vi "grabber fpga details panel.vi"() -> ()   [LabVIEW 2010]
uses:
  scan_specification_tagResonant.ctl
  common_typedefs/DAC_voltage_tagResonantr.ctl
  counter_cluster_tagResonant.ctl
  FPGA_ref.ctl
  <vilib>/Platform/TimedLoop/XDataNode/XDataNode.xnode
  <vilib>/Platform/TimedLoop/XDataNode/timing_clust.ctl
  <vilib>/Platform/TimedLoop/XDataNode/nitl_modes.ctl
  <vilib>/Platform/TimedLoop/XDataNode/wakeup.ctl
  <vilib>/rvi/interface/nirviReadWriteControl/nirviReadWriteControl.xnode
  <vilib>/rvi/interface/common/niFpgaNodeNameForErrorReporting.ctl
  <vilib>/rvi/errors/niLvFpgaWhatHappensToTopLevelVI.ctl
  <vilib>/Utility/error.llb/Error Cluster From Error Code.vi
  <vilib>/rvi/errors/niLvFpgaAdjustHostInterfaceError.vi
  <vilib>/Platform/TimedLoop/XDataNode/XDNodeRunTimeDep.lvlib
  NiFpgaLv.dll
panel:
  out "z-location":i16
  out "z state.pos estimate":fxp<+/-,32,16> format="%.21g"
  out "piezo z-offset":i16
  out "piezo out":i16
  in  "FPGARef":T1
  out "counter cluster out":T2
  out "scanning? FPGA":bool
  out "scan":bool
  out "FIFO overflow":bool
  out "acquire?":bool
  out "DAC voltages":T3 {"pockels" max=4095 step=1; "y" max=4095 step=1; "x" max=4095 step=1}
  out "scan specification":T4={"z resolution (pixels)"=100, "iterations per pixel"=28, "iterations per z-scan (=zres*iterperpixel)"=50, "x resolution (pixels)"=100, "y resolution (pixels)"=80, "number of z-lines per volume"=30, "number of repetitions (volumes)"=5, "Pockels cell voltage (bits)"=80, "Vx center (bits)"=0, "Vy center (bits)"=0, "Vx amplitude (bits)"=40, "Vy amplitude (bits)"=0, "lines to delay between scan start and output"=1, "LSB has acquire control"=FALSE}
  out "fpga command loop info":T5
  out "pixels acquired-1":u64
  out "lines sent":u32
  out "pixels sent":u32
  in  "stop":bool
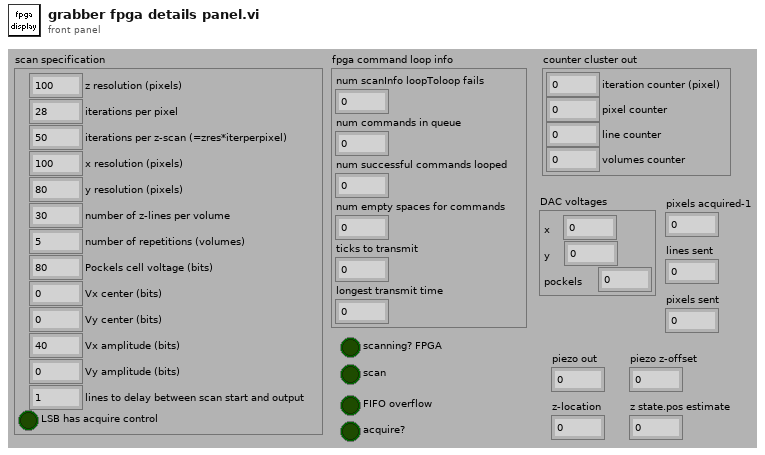
[diagram p1: front panel]
types:
  T1 = typedef "FPGA_ref.ctl" = refnum<k20>
  T2 = typedef "counter_cluster_tagResonant.ctl" = cluster{"iteration counter (pixel)":u16, "pixel counter":u16, "line counter":i16, "volumes counter":u16}
  T3 = typedef "DAC_voltage_tagResonantr.ctl" = cluster{"x":i16, "y":i16, "pockels":i16}
  T4 = typedef "scan_specification_tagResonant.ctl" = cluster{"z resolution (pixels)":u16, "iterations per pixel":u16, "iterations per z-scan (=zres*iterperpixel)":u16, "x resolution (pixels)":u16, "y resolution (pixels)":u16, "number of z-lines per volume":u16, "number of repetitions (volumes)":i32, "Pockels cell voltage (bits)":i16, "Vx center (bits)":i16, "Vy center (bits)":i16, "Vx amplitude (bits)":i16, "Vy amplitude (bits)":i16, "lines to delay between scan start and output":u16, "LSB has acquire control":bool}
  T5 = cluster{"num scanInfo loopToloop fails":u32, "num commands in queue":u32, "num successful commands looped":u32, "num empty spaces for commands":u32, "ticks to transmit":i32, "longest transmit time":i32}
  T6 = typedef "XDNodeRunTimeDep.lvlib/timing_clust.ctl" = cluster{"Expected End [f-1]":u64, "Actual End [f-1]":u64, "Finished Late? [f-1]":bool, "Expected End [i-1]":u64, "Actual End [i-1]":u64, "Finished Late? [i-1]":bool, "Expected Start [i]":u64, "Actual Start [i]":u64, "Expected Start [f]":u64, "Actual Start [f]":u64, "Source Name":string, "Structure Name":string, "Period":i64, "Deadline":i64, "Offset":i64, "Start":i64, "Priority":i32, "Timeout":i32, "Mode":T7, "Wakeup Reason":T8, "Error":errorcluster, "Source Type":string, "Secondary Source Type":string, "Global End Time":u64, "Global Start Time":u64, "Frame Duration":u64, "Iteration Duration":u64, "Assigned CPU":i32, "I/O Scan Engine Mode":u32}
  T7 = typedef "XDNodeRunTimeDep.lvlib/nitl_modes.ctl" = enum32{"No Change", "Process missed periods, maintain original phase", "Discard missed periods, maintain original phase", "Process missed periods, ignore original phase", "Discard missed periods, ignore original phase"}
  T8 = typedef "XDNodeRunTimeDep.lvlib/wakeup.ctl" = enum32{"Normal", "Aborted", "Asynchronous wakeup", "Timing source error", "Timed loop error", "Timeout"}
  T9 = cluster{"x state":cluster{"pos estimate":fxp<+/-,32,16>, "v estimate":fxp<+/-,16,0>, "weighted position error sum":fxp<+/-,32,32>, "photon count":u32, "transmit tick count":u32, "axis number":u8, "px (levels^2)":fxp<+,32,19>, "pxv (levels^2/ticks)":fxp<+,32,2>, "pv (levels^2/ticks^2)":fxp<+,32,-14>, "vel diff (levels^2/ticks^3)":fxp<+,24,-22>, "gx":fxp<+,16,8>, "rtwiddle":fxp<+,16,26>, "photon count ch0":u32, "photon count ch1":u32, "Dx - for pos only k-f":fxp<+,32,19>}, "y state":cluster{"pos estimate":fxp<+/-,32,16>, "v estimate":fxp<+/-,16,0>, "weighted position error sum":fxp<+/-,32,32>, "photon count":u32, "transmit tick count":u32, "axis number":u8, "px (levels^2)":fxp<+,32,19>, "pxv (levels^2/ticks)":fxp<+,32,2>, "pv (levels^2/ticks^2)":fxp<+,32,-14>, "vel diff (levels^2/ticks^3)":fxp<+,24,-22>, "gx":fxp<+,16,8>, "rtwiddle":fxp<+,16,26>, "photon count ch0":u32, "photon count ch1":u32, "Dx - for pos only k-f":fxp<+,32,19>}, "z state":cluster{"pos estimate":fxp<+/-,32,16>, "v estimate":fxp<+/-,16,0>, "weighted position error sum":fxp<+/-,32,32>, "photon count":u32, "transmit tick count":u32, "axis number":u8, "px (levels^2)":fxp<+,32,19>, "pxv (levels^2/ticks)":fxp<+,32,2>, "pv (levels^2/ticks^2)":fxp<+,32,-14>, "vel diff (levels^2/ticks^3)":fxp<+,24,-22>, "gx":fxp<+,16,8>, "rtwiddle":fxp<+,16,26>, "photon count ch0":u32, "photon count ch1":u32, "Dx - for pos only k-f":fxp<+,32,19>}}
  T10 = cluster{"iteration counter (pixel)":u16, "pixel counter":u16, "line counter":i16, "volumes counter":u16}
  T11 = cluster{"z resolution (pixels)":u16, "iterations per pixel":u16, "iterations per z-scan (=zres*iterperpixel)":u16, "x resolution (pixels)":u16, "y resolution (pixels)":u16, "number of z-lines per volume":u16, "number of repetitions (volumes)":i32, "Pockels cell voltage (bits)":i16, "Vx center (bits)":i16, "Vy center (bits)":i16, "Vx amplitude (bits)":i16, "Vy amplitude (bits)":i16, "lines to delay between scan start and output":u16, "LSB has acquire control":bool}
  T12 = typedef "niFpgaNodeNameForErrorReporting.ctl" = enum16{"Open FPGA VI Reference", "Read/Write Control", "Invoke Method: Abort", "Invoke Method: Acknowledge IRQ", "Invoke Method: Download", "Invoke Method: FIFO.Configure", "Invoke Method: FIFO.Read", "Invoke Method: FIFO.Start", "Invoke Method: FIFO.Stop", "Invoke Method: FIFO.Write", "Invoke Method: Reset", "Invoke Method: Run", "Invoke Method: Wait on IRQ", "Close FPGA VI Reference"}
  T13 = typedef "niLvFpgaWhatHappensToTopLevelVI.ctl" = enum16{"top level VI scripted behind XNode", "top level VI inlined behind XNode"}
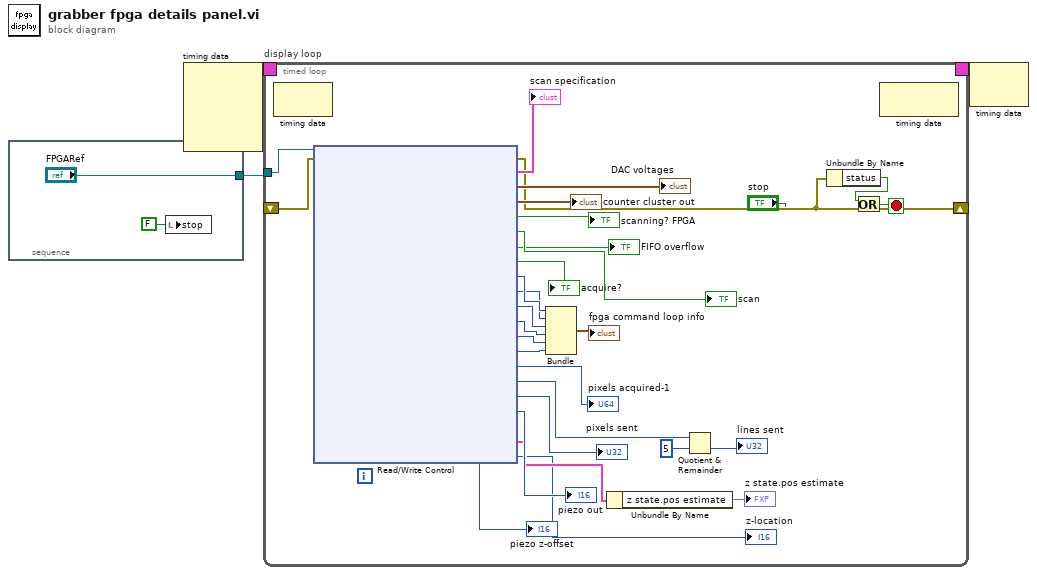
[diagram p0: block diagram]
diagram:
  n1 = stacked-sequence {
    tunnel: ["FPGARef"] -> w1
    frame #0 {
      n2 = local write "stop"(FALSE ("stop")) -> ()
    }
  }
  n3 = node-c288() -> (w3:T6)  [unwired: 4 in]
  n4 = timed-loop "display loop" {
    shift-right: [w14] -> _
    shift-left: _ -> [w15]
    timing: w3 -> [_]
    timing-out: [_] -> w2
    tunnel: w1 -> [w16]
    stop <- w35 stop-if-true
    n5 = node-c288() -> ()  [unwired: 1 in, 1 out]
    n6 = xnode "Read/Write Control"("FPGA VI Reference In"=w16, "error in"=w15) -> ("error out"=w14:errorcluster, "scan specification"=→"scan specification":T11, "DAC voltages"=→"DAC voltages":cluster{"x":i16, "y":i16, "pockels":i16}, "counter cluster out"=→"counter cluster out":T10, "scanning?"=→"scanning? FPGA":bool, "scan"=→"scan":bool, "FIFO overflow"=→"FIFO overflow":bool, "acquire?"=→"acquire?":bool, "num scanInfo loopToloop fails"=w29:u32, "num commands in queue"=w28:u32, "num successful commands looped"=w27:u32, "num empty spaces for commands"=w26:u32, "ticks to transmit"=w25:i32, "longest transmit time"=w24:i32, "pixels acquired-1"=→"pixels acquired-1":u64, "lines sent"=w19:u32, "pixels sent"=→"pixels sent":u32, "piezo out"=→"piezo out":i16, "piezo z-offset"=→"piezo z-offset":i16, "kalman state"=w8:T9, "z-location"=→"z-location":i16)  [unwired: 1 out]
    n7 = Bundle("num scanInfo loopToloop fails"=w29, "num commands in queue"=w28, "num successful commands looped"=w27, "num empty spaces for commands"=w26, "ticks to transmit"=w25, "longest transmit time"=w24) -> (→"fpga command loop info":T5)  [unwired: 1 in]
    n8 = Unbundle By Name(w8) -> ("z state.pos estimate"=→"z state.pos estimate":fxp<+/-,32,16>)
    n9 = Quotient & Remainder(x=w19, y=u32 5) -> (floor(x/y)=→"lines sent":u32)  [unwired: 1 out]
    n10 = Unbundle By Name(w14) -> ("status"=w13:bool)
    n11 = Or(x=w13, y="stop") -> (x .or. y?=w35:bool)
    n12 = node-c288() -> ()  [unwired: 1 in, 1 out]
  }
  n13 = node-c288(w2) -> ()  [unwired: 1 out]
